vi "Configure Limit Test Table.vi"(0 "VISA resource name":refnum<visa-resource-name>, 1 "Number of Lines (0)":i32, 2 "Type of Line (0)":i32[](array[numeric]), 5 "Channel (1)":i32=1, 7 "Start Point X Value (0.0)":dbl[](array[numeric]), 9 "End Point X Value (0.0)":dbl[](array[numeric]), 11 "error in (no error)":errorcluster, 12 "Start Point Y Value (0.0)":dbl[](array[numeric]), 13 "End Point Y Value (0.0)":dbl[](array[numeric])) -> (4 "VISA resource name out":refnum<visa-resource-name>, 15 "error out":errorcluster)   [LabVIEW 2018, in "Agilent ENA Series.lvlib"]
doc: "Configures the limit table."
uses:
  Agilent ENA Series.lvlib
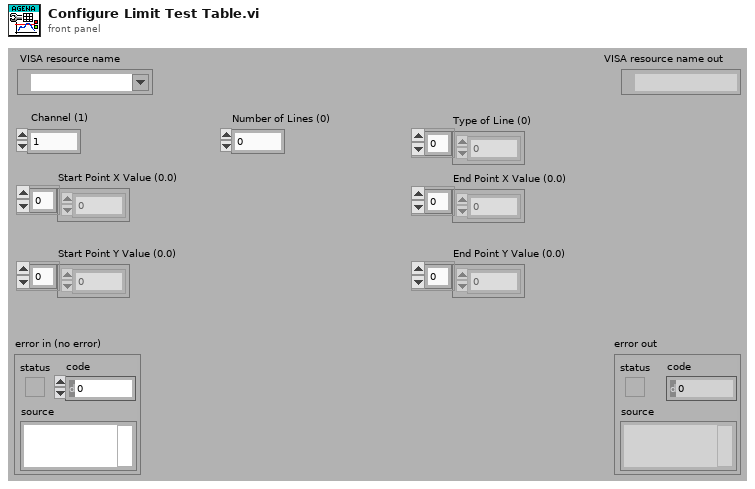
[diagram p1: front panel]
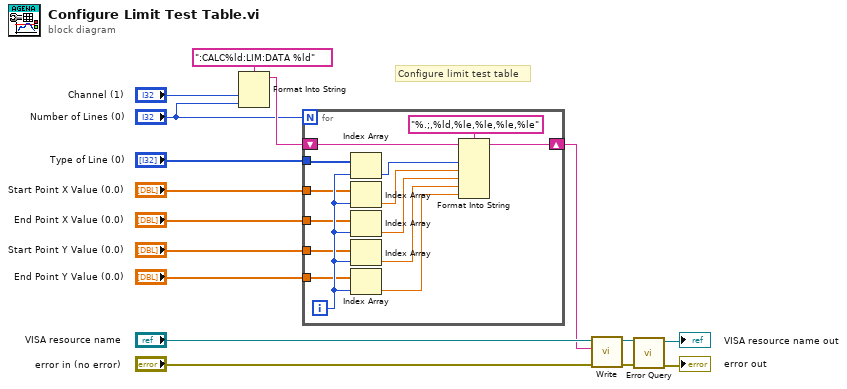
[diagram p0: block diagram]
diagram:
  # "Configure limit test table"
  n1 = Format Into String(format string=":CALC%ld:LIM:DATA %ld", "Channel (1)", "Number of Lines (0)") -> (resulting string=w12:string)  [unwired: 2 in, 1 out]
  n2 = for {
    N: "Number of Lines (0)" -> [_]
    shift-right: [w28] -> w6
    shift-left: w12 -> [w29]
    tunnel: "Type of Line (0)" -> [w22]
    tunnel: "Start Point X Value (0.0)" -> [w23]
    tunnel: "End Point X Value (0.0)" -> [w24]
    tunnel: "Start Point Y Value (0.0)" -> [w25]
    tunnel: "End Point Y Value (0.0)" -> [w26]
    i -> [w27]
    n3 = Index Array(array=w22, index=w27) -> (element=w21:i32)
    n4 = Index Array(array=w23, index=w27) -> (element=w20:dbl)
    n5 = Index Array(array=w24, index=w27) -> (element=w19:dbl)
    n6 = Index Array(array=w25, index=w27) -> (element=w18:dbl)
    n7 = Index Array(array=w26, index=w27) -> (element=w17:dbl)
    n8 = Format Into String(format string="%.;,%ld,%le,%le,%le,%le", initial string=w29, w21, w20, w19, w18, w17) -> (resulting string=w28:string)  [unwired: 1 in, 1 out]
  }
  n9 = call "Write.vi"("error in (no error)"="error in (no error)", "String ()"=w6, "VISA resource name"="VISA resource name") -> ("error out"=w3:errorcluster, "VISA resource name out"=w4:refnum<visa-resource-name>)  [unwired: 6 in, 1 out]
  n10 = call "Error Query.vi"("error in (no error)"=w3, "VISA resource name"=w4) -> ("error out"=→"error out":errorcluster, "VISA resource name out"=→"VISA resource name out":refnum<visa-resource-name>)  [unwired: 6 in, 2 out]
